vi "SDSU_DAC_GetResolution.vi"(10 "resolutions":string[][](table), 11 "type":string) -> (2 "max counts":i32)   [LabVIEW 2016]
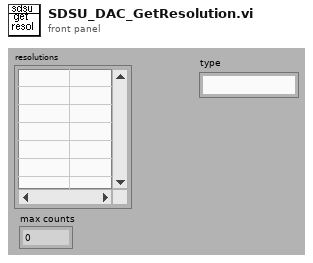
[diagram p1: front panel]
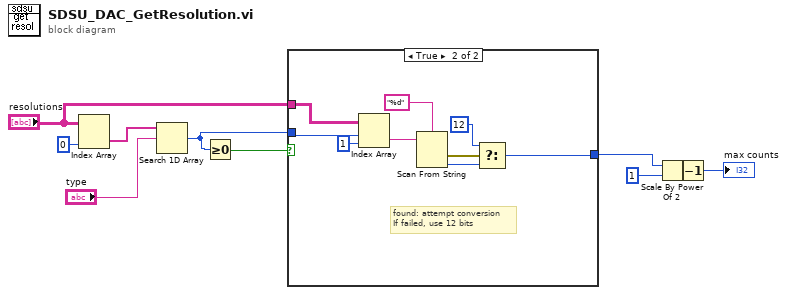
[diagram p0: block diagram]
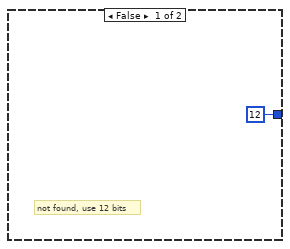
[diagram p2: hidden frame]
diagram:
  n1 = Index Array(array="resolutions", index (col)=0 ("disabled index (col)")) -> (element=w9:string[])  [unwired: 1 in]
  n2 = Search 1D Array(1D array=w9, element="type") -> (index of element=w6:i32)  [unwired: 1 out]
  n3 = Greater Or Equal To 0?(x=w6) -> (x >= 0?=w7:bool)
  n4 = case shown="True" w7 {
    tunnel: w6 -> [_ w19]
    tunnel: "resolutions" -> [_ w20]
    tunnel: [12 ("t") w12] -> w2
    frame False {
      # "not found, use 12 bits"
    }
    frame True {
      # "found: attempt conversion\nIf failed, use 12 bits"
      n5 = Index Array(array=w20, index (row)=w19, index (col)=1 ("disabled index (col)")) -> (element=w16:string)
      n6 = Scan From String(format string="%d", input string=w16) -> (error out=w15:errorcluster, output 1=w14:i32)  [unwired: 2 in, 3 out]
      n7 = Select(t=12, s=w15, f=w14) -> (s? t:f=w12:i32)
    }
  }
  n8 = Scale By Power Of 2(n=w2, x=1) -> (x*2^n=w3:i32)
  n9 = Decrement(x=w3) -> (x-1=→"max counts":i32)
